vi "Get refnum.vi"(8 "Error In":errorcluster, 11 "MDI.lvlib:Document.lvclass":refnum<class "Document.lvclass">) -> (0 "Error Out":errorcluster, 1 "VI Refnum":refnum<vi>, 3 "MDI.lvlib:Document.lvclass 2":refnum<class "Document.lvclass">)   [LabVIEW 2016, in "Document.lvclass"]
uses:
  Document.lvclass
  Document.lvclass/Document.ctl
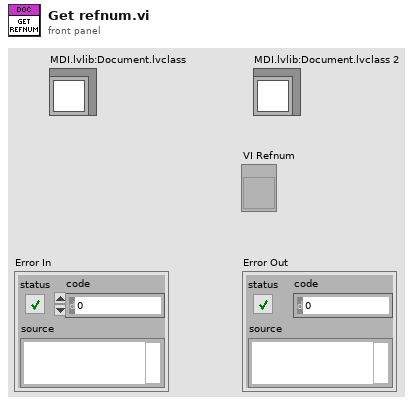
[diagram p1: front panel]
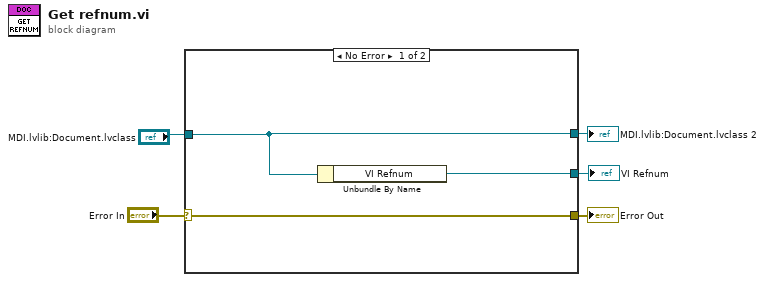
[diagram p0: block diagram]
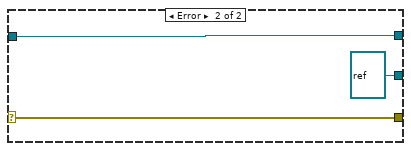
[diagram p2: hidden frame]
diagram:
  n1 = case shown="No Error" "Error In" {
    selector: "Error In" -> [w8 w11]
    tunnel: [w8 w11] -> w4
    tunnel: "MDI.lvlib:Document.lvclass" -> [w7 w10]
    tunnel: [w7 w10] -> w2
    tunnel: [w6 refnum<vi> refnum ("VI Refnum")] -> w1
    frame No Error {
      n2 = Unbundle By Name(w7) -> ("VI Refnum"=w6:refnum<vi>)
    }
    frame Error {
    }
  }
  "Error Out" <- w4
  "MDI.lvlib:Document.lvclass 2" <- w2
  "VI Refnum" <- w1
